vi "ConvertToPartyModeCommand.vi"(10 "Device Name":string, 11 "Command":string) -> (3 "Command out":string)   [LabVIEW 2015]
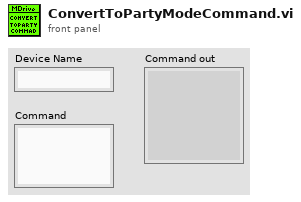
[diagram p1: front panel]
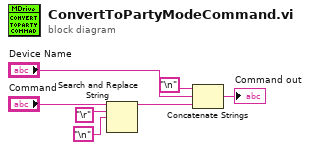
[diagram p0: block diagram]
diagram:
  n1 = Search and Replace String(input string="Command", search string="\r", replace string="\n") -> (result string=w6:string)  [unwired: 5 in, 3 out]
  n2 = Concatenate Strings("\n", "Device Name", w6) -> (→"Command out":string)
